vi "Torque Input and Output.vi"() -> ()   [LabVIEW 2019, in "Part of Main VIs.lvlib" / "Torque Library.lvlib"]
uses:
  Torque Library.lvlib
  <vilib>/Utility/error.llb/DialogType.ctl
  <extravilib>/ChannelInstances/Tag-str/Read With Abort.vi
  <extravilib>/ChannelInstances/Tag-dbl/Read With Abort.vi
  <extravilib>/ChannelInstances/Tag-str/Write With Abort.vi
  <extravilib>/ChannelInstances/Tag-dbl/Write With Abort.vi
  <extravilib>/ChannelInstances/Tag-str/Instantiate.vi
  <extravilib>/ChannelInstances/Tag-str/EndpointRead.vi
  <extravilib>/ChannelInstances/Tag-dbl/Instantiate.vi
  <extravilib>/ChannelInstances/Tag-dbl/EndpointRead.vi
  <extravilib>/ChannelInstances/Tag-str/Endpoint.vi
  <extravilib>/ChannelInstances/Tag-dbl/Endpoint.vi
  Torque VI.lvlib
  <extravilib>/ChannelInstances/Tag-dbl.lvlib
  <extravilib>/ChannelInstances/Tag-str.lvlib
  Command VI.lvlib
panel:
  out "Analog Input Logging Path":path
  out "String 2":string
  in  "String":string
  out "Waveform Chart":waveform(dbl)(graph)
  in  "Numeric":dbl
  out "Analog DC Voltage":waveform(dbl)(graph)
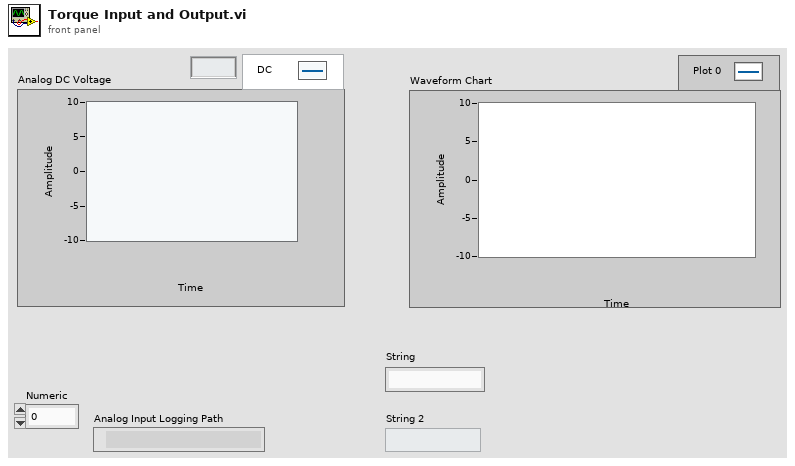
[diagram p1: front panel]
types:
  T1 = typedef "DialogType.ctl" = u16
  T2 = typedef "Tag-str.lvlib/))Channel.ctl" = refnum<queue>
  T3 = typedef "Tag-dbl.lvlib/))Channel.ctl" = refnum<queue>
  T4 = enum16{"open", "replace", "create", "open or create", "replace or create", "replace or create with confirmation"}
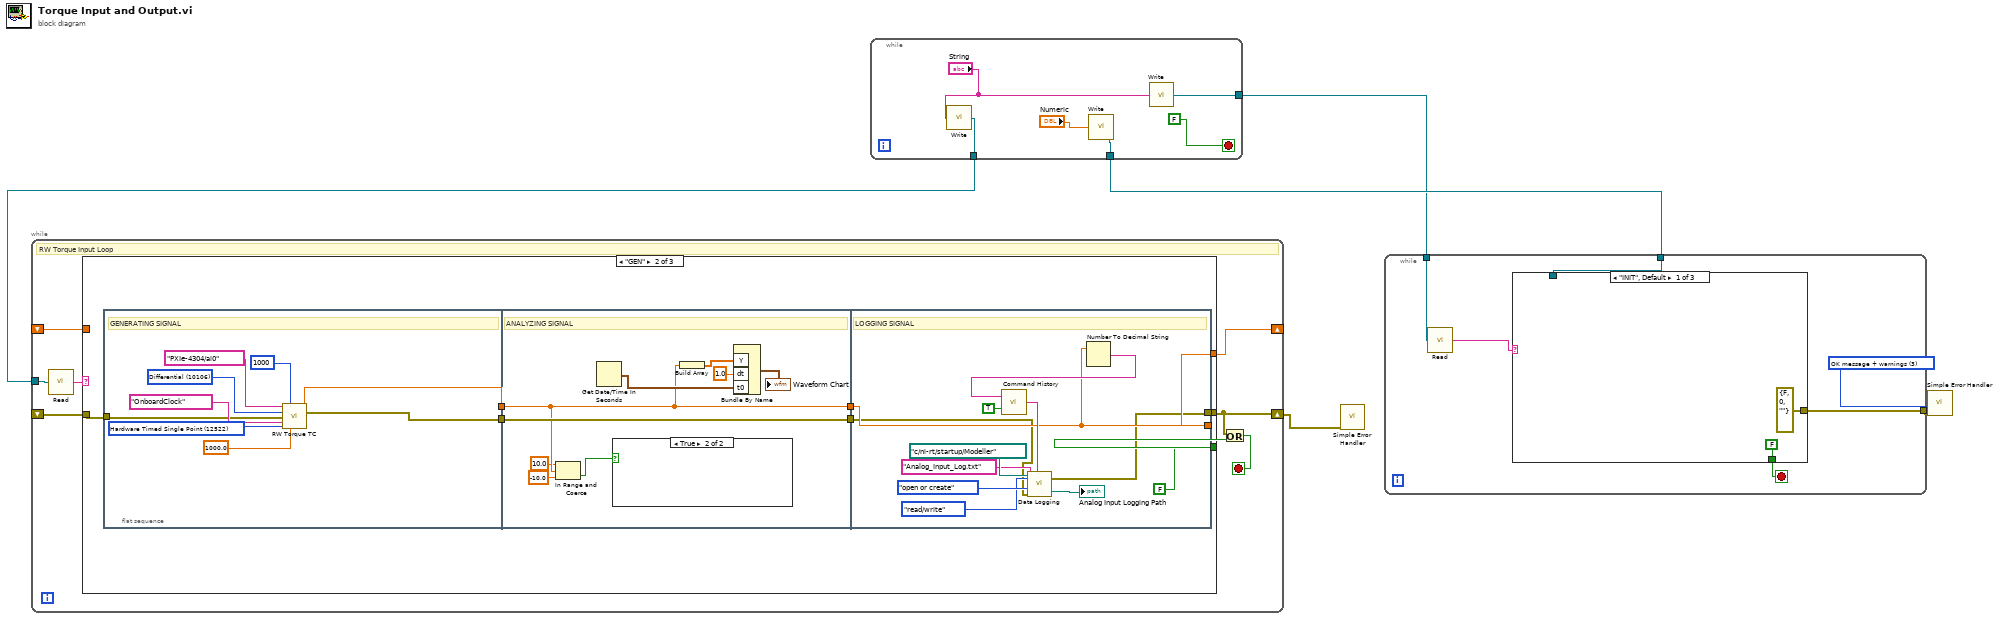
[diagram p0: block diagram]
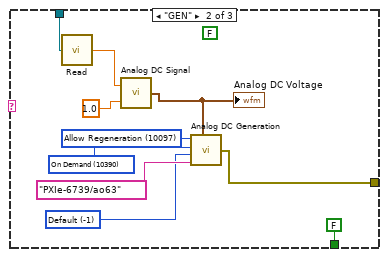
[diagram p2: hidden frame]
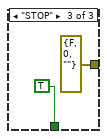
[diagram p3: hidden frame]
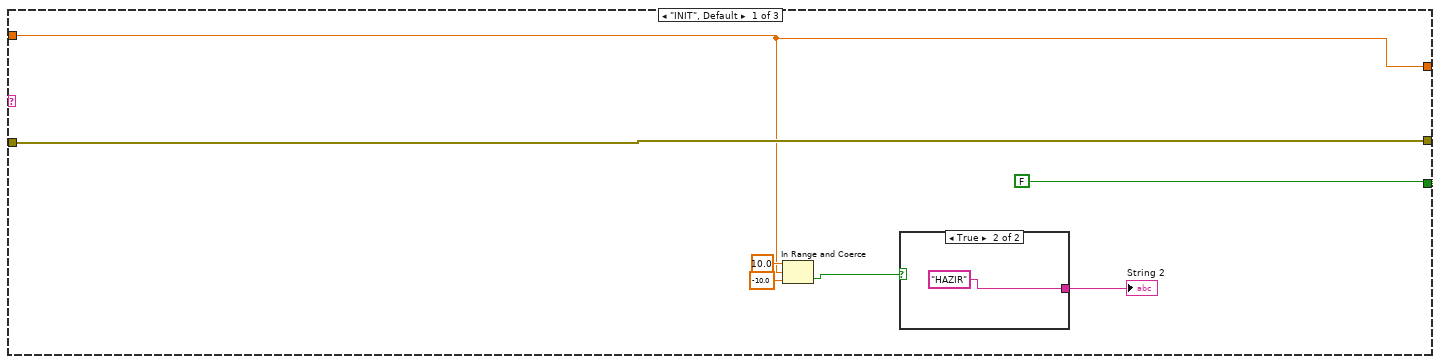
[diagram p4: hidden frame]
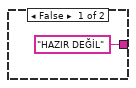
[diagram p5: hidden frame]
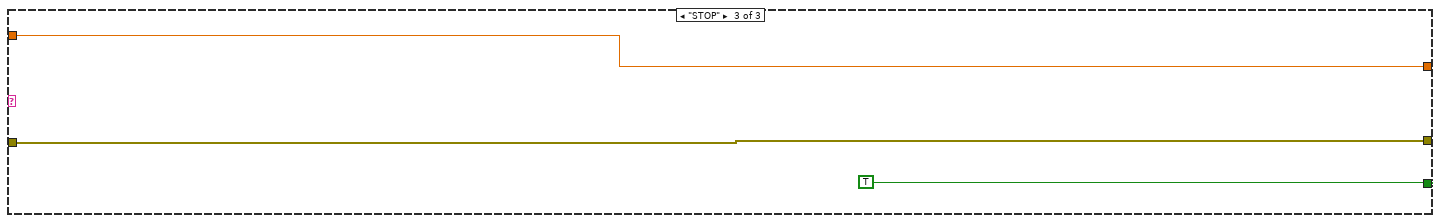
[diagram p7: hidden frame]
diagram:
  w6 = T1 3 items=["no dialog", "OK message", "continue or stop message", "OK message + warnings", "continue/stop + warnings"] ("type of dialog (OK msg:1)")
  n1 = while {
    tunnel: [w11] -> w4
    tunnel: [w10] -> w2
    tunnel: [w8] -> w3
    stop <- FALSE stop-if-true
    n2 = call <extravilib>:"Write.vi"("element"="String") -> ("channel"=w10:T2)  [unwired: 1 out]
    n3 = call <extravilib>:"Write.vi"("element"="Numeric") -> ("channel"=w11:T3)  [unwired: 1 out]
    n4 = call <extravilib>:"Write.vi"("element"="String") -> ("channel"=w8:T2)  [unwired: 1 out]
  }
  n5 = while {
    shift-right: [w13] -> w1
    shift-left: _ -> [w20]
    shift-right: [w16] -> _
    shift-left: _ -> [w17]
    tunnel: w2 -> [w15]
    stop <- w18 stop-if-true
    # "RW Torque Input Loop"
    n6 = call <extravilib>:"Read.vi"("channel"=w15) -> ("element"=w14:string)  [unwired: 1 in, 1 out]
    n7 = case shown="\"GEN\"" w14 {
      tunnel: w20 -> [w26 w33 w69]
      tunnel: [w26 w31 w69] -> w13
      tunnel: [FALSE FALSE TRUE] -> w19
      tunnel: [w21 w34 w67] -> w16
      tunnel: w17 -> [w21 _ w67]
      frame "INIT", Default {
        n8 = In Range and Coerce(upper limit=10.0, x=w21, lower limit=-10.0) -> (In Range?=w25:bool)  [unwired: 1 out]
        n9 = case shown="True" w25 {
          tunnel: ["HAZIR DEĞİL" ("String 2") "HAZIR" ("String 2")] -> w22
          frame False {
          }
          frame True {
          }
        }
        "String 2" <- w22
      }
      frame "GEN" {
        n10 = flat-sequence {
          tunnel: [w40] -> w36
          tunnel: w33 -> [w38]
          tunnel: [w39] -> w32
          tunnel: w36 -> [w50]
          tunnel: [w50] -> w35
          tunnel: w32 -> [w51]
          tunnel: [w51] -> w30
          tunnel: w35 -> [w58]
          tunnel: [w58] -> w34
          tunnel: [w57] -> w31
          tunnel: w30 -> [w56]
          frame #0 {
            w42 = 12522 items=["Finite Samples"=10178, "Continuous Samples"=10123, "Hardware Timed Single Point"=12522] ("sample mode")
            w44 = 10106 items=["Default"=-1, "RSE"=10083, "NRSE"=10078, "Differential"=10106, "Pseudodifferential"=12529] ("input terminal configuration")
            # "GENERATING SIGNAL"
            n11 = call "RW Torque TC.vi"("physical channels"=tag "PXIe-4304/ai0", "samples per channel"=1000, "input terminal configuration"=w44, "error in"=w38, "source"=tag "OnboardClock", "sample mode"=w42, "rate"=1000.0) -> ("data"=w40:dbl, "error out"=w39:errorcluster)  [unwired: 7 in]
          }
          frame #1 {
            # "ANALYZING SIGNAL"
            n12 = In Range and Coerce(upper limit=10.0, x=w50, lower limit=-10.0) -> (In Range?=w47:bool)  [unwired: 1 out]
            n13 = Get Date/Time In Seconds() -> (seconds since 1Jan1904=w55:timestamp)
            n14 = case shown="True" w47 {
              frame False {
              }
              frame True {
              }
            }
            n15 = Build Array(w50) -> (w53:dbl[])
            n16 = Bundle By Name("Y"=w53, "dt"=1.0, "t0"=w55) -> (→"Waveform Chart":waveform(dbl))  [unwired: 1 in]
          }
          frame #2 {
            # "LOGGING SIGNAL"
            n17 = Number To Decimal String(number=w58) -> (decimal integer string=w59:string)  [unwired: 1 in]
            n18 = call "Command History.vi"("want seconds? (F)"=TRUE, "Command from UDP"=w59) -> ("Command History"=w61:string)
            n19 = call "Data Logging.vi"("text"=w61, "access (0:read/write)"=enum16{"read/write", "read-only", "write-only"}."read/write", "error in"=w56, "operation (0:open)"=T4."open or create", "file"="Analog_Input_Log.txt", "path"=path "c:/ni-rt/startup/Modeller") -> ("path"=→"Analog Input Logging Path":path, "error out"=w57:errorcluster)
          }
        }
      }
      frame "STOP" {
      }
    }
    n20 = Or(x=w13, y=w19) -> (x .or. y?=w18:bool)
  }
  n21 = call <vilib>:"Simple Error Handler.vi"("error in (no error)"=w1) -> ()  [unwired: 4 in, 5 out]
  n22 = while {
    tunnel: [w74] -> w5
    tunnel: w4 -> [w73]
    tunnel: w3 -> [w71]
    stop <- w72 stop-if-true
    n23 = call <extravilib>:"Read.vi"("channel"=w71) -> ("element"=w70:string)  [unwired: 1 in, 1 out]
    n24 = case shown="\"INIT\", Default" w70 {
      tunnel: [errorcluster {"status"=FALSE, "code"=0, "source"=""} ("error out") w81 errorcluster {"status"=FALSE, "code"=0, "source"=""} ("error out")] -> w74
      tunnel: w73 -> [_ w79 _]
      tunnel: [FALSE FALSE TRUE] -> w72
      frame "INIT", Default {
      }
      frame "GEN" {
        (unwired) FALSE
        w82 = -1 items=["Default"=-1, "RSE"=10083, "Differential"=10106, "Pseudodifferential"=12529] ("output terminal configuration")
        w84 = 10390 items=["Sample Clock"=10388, "Burst Handshake"=12548, "Handshake"=10389, "Implicit"=10451, "On Demand"=10390, "Change Detection"=12504, "Pipelined Sample Clock"=14668] ("SampTimingType")
        w85 = 10097 items=["Allow Regeneration"=10097, "Do Not Allow Regeneration"=10158] ("RegenMode")
        n25 = call <extravilib>:"Read.vi"("channel"=w79) -> ("element"=w78:dbl)  [unwired: 1 in, 1 out]
        n26 = call "Analog DC Signal.vi"("dt"=1.0, "Amplitude"=w78) -> ("DC Analog Signal"=w80:waveform(dbl))
        "Analog DC Voltage" <- w80
        n27 = call "Analog DC Generation.vi"("RegenMode"=w85, "SampTimingType"=w84, "output terminal configuration"=w82, "physical channels"=tag "PXIe-6739/ao63", "data"=w80) -> ("error out"=w81:errorcluster)
      }
      frame "STOP" {
      }
    }
  }
  n28 = call <vilib>:"Simple Error Handler.vi"("type of dialog (OK msg:1)"=w6, "error in (no error)"=w5) -> ()  [unwired: 3 in, 5 out]
